vi "Set Last Waveforms.vi"(8 "Error In":errorcluster, 10 "Last Waveforms":map{u8, waveform(dbl)}(c390), 11 "reference in":refnum<class "Scope Base.lvclass">) -> (0 "Error Out":errorcluster, 3 "reference out":refnum<class "Scope Base.lvclass">)   [LabVIEW 2023, in "Scope Base.lvlib" / "Scope Base.lvclass"]
uses:
  Scope Base.lvclass
  Scope Base.lvclass/Scope Base.ctl
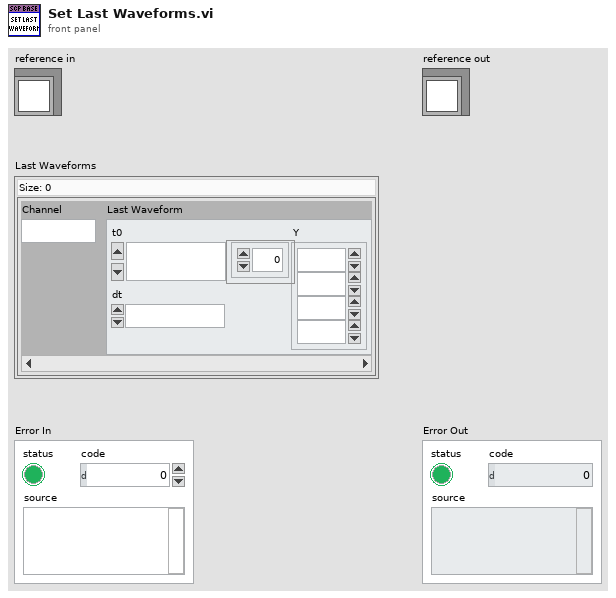
[diagram p1: front panel]
types:
  T1 = typedef "Scope Base.lvlib/Scope Base.lvclass/ObjectAttributes.ctl" = cluster{"Last Waveforms":map{u8, waveform(dbl)}}
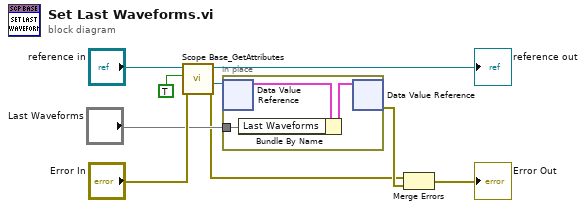
[diagram p0: block diagram]
diagram:
  n1 = call "Scope Base_GetAttributes.vi"("Error In"="Error In", "OnlyGetDvrReference(False)"=TRUE, "reference in"="reference in") -> ("Error Out"=w3:errorcluster, "DataRef"=w1:refnum<data-value>, "reference out"=→"reference out":refnum<class "Scope Base.lvclass">)  [unwired: 5 in, 1 out]
  n2 = in-place {
    in-place-border: "Last Waveforms" -> [w10]
    n3 = in-place-dvr #1(w1) -> (w12:T1)  [unwired: 1 out]
    n4 = Bundle By Name(cluster=w12, "Last Waveforms"=w10) -> (w11:T1)
    n5 = in-place-dvr #1(w11) -> (w4:errorcluster)  [unwired: 1 out]
  }
  n6 = Merge Errors(w3, w4) -> (→"Error Out":errorcluster)
